vi "PPMS Global.vi"() -> ()   [LabVIEW 2013]
panel:
  out "Helium Level String":string
  out "Helium Level":dbl=100.0
  out "Rate (K/min)":dbl=5.0
  out "Rate (Oe/s)":dbl=10.0
  out "Target Position":dbl
  out "Target Temp":dbl
  out "Target Field":dbl
  out "Set Position?":bool
  out "Set Temp?":bool
  out "Set Field?":bool
  out "Position (Degree)":dbl=-0.001072365790605545
  out "PPMS IP Address":string="130.49.180.87"
  out "Field (Oe)":dbl=-0.001072365790605545
  out "Temperature (K)":dbl=309.9967
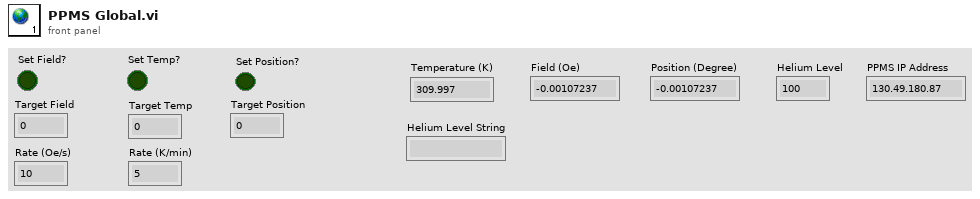
[diagram p1: front panel]
diagram:
